vi "date and time info.vi"() -> (3 "Output String":string)   [LabVIEW 2014]
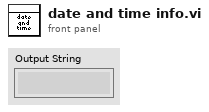
[diagram p1: front panel]
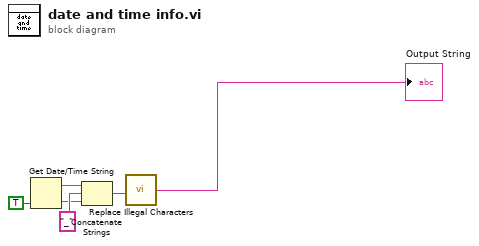
[diagram p0: block diagram]
diagram:
  n1 = Get Date/Time String(want seconds? (F)=TRUE) -> (date string=w3:string, time string=w2:string)  [unwired: 2 in]
  n2 = Concatenate Strings(w3, "_" ("string"), w2) -> (w4:string)
  n3 = call "Replace Illegal Characters.vi"("String"=w4) -> ("Output String"=→"Output String":string)  [unwired: 2 in]
